vi "Solve2.vi"(8 "Error In":errorcluster, 11 "object in":refnum<class "2021_7.lvclass">) -> (0 "Error Out":errorcluster, 2 "Result":u64, 3 "object out":refnum<class "2021_7.lvclass">)   [LabVIEW 2020, in "2021_7.lvclass"]
uses:
  2021_7.lvclass
  2021_7.lvclass/2021_7.ctl
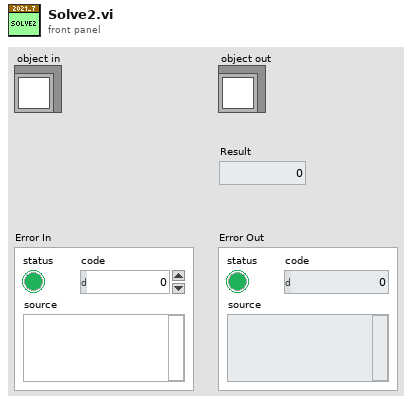
[diagram p1: front panel]
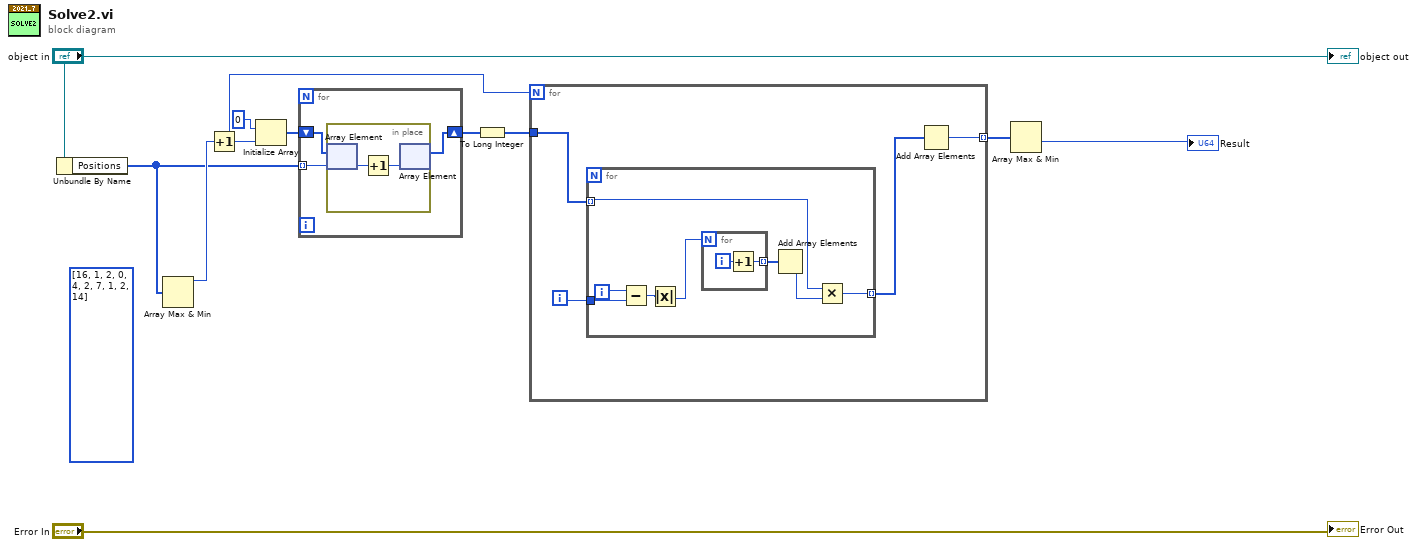
[diagram p0: block diagram]
diagram:
  (unwired) i32[] [16, 1, 2, 0, 4, 2, 7, 1, 2, 14] ("FishTimers")
  n1 = Unbundle By Name("object in") -> ("Positions"=w1:u32[])
  n2 = Array Max & Min(array=w1) -> (max value=w7:u32)  [unwired: 3 out]
  n3 = Increment(x=w7) -> (x+1=w5:u32)
  n4 = Initialize Array(u64 0 ("new element/subarray"), w5) -> (w8:u64[])
  n5 = for {
    tunnel: w1 -> [w13] mode=indexing
    shift-right: [w12] -> w6
    shift-left: w8 -> [w14]
    n6 = in-place {
      n7 = in-place-array #1(w14, w13) -> (w16:u64)
      n8 = Increment(x=w16) -> (x+1=w15:u64)
      n9 = in-place-array #1(w15) -> (w12:u64[])  [unwired: 1 out]
    }
  }
  n10 = To Long Integer(number=w6) -> (32bit integer=w4:i32[])
  n11 = for {
    N: w5 -> [_]
    tunnel: w4 -> [w19]
    tunnel: [w20] -> w3 mode=indexing
    i -> [w18]
    n12 = for {
      tunnel: w19 -> [w24] mode=indexing
      tunnel: w18 -> [w27]
      tunnel: [w25] -> w17 mode=indexing
      i -> [w28]
      n13 = Subtract(x=w28, y=w27) -> (x-y=w26:i32)
      n14 = Absolute Value(x=w26) -> (abs(x)=w22:i32)
      n15 = for {
        N: w22 -> [_]
        tunnel: [w29] -> w23 mode=indexing
        i -> [w30]
        n16 = Increment(x=w30) -> (x+1=w29:i32)
      }
      n17 = Add Array Elements(numeric array=w23) -> (sum=w21:i32)
      n18 = Multiply(x=w24, y=w21) -> (x*y=w25:i32)
    }
    n19 = Add Array Elements(numeric array=w17) -> (sum=w20:i32)
  }
  n20 = Array Max & Min(array=w3) -> (min value=→"Result":i32)  [unwired: 3 out]
  "Error Out" <- "Error In"
  "object out" <- "object in"
